vi "Fingerprint Length.vi"(8 "Error In":errorcluster) -> (0 "Error Out":errorcluster)   [LabVIEW 2017, in "Tests.lvlib" / "Session.lvlib"]
uses:
  Session.lvlib
  src/Toolkit/API/Session/API/Typedefs/Host Key Hash Types.ctl
  <vilib>/addons/_JKI Toolkits/Caraya/classes/Test/Test.lvclass
  src/Toolkit/Toolkit.lvlib
  src/Toolkit/API/Session/Session.lvclass
  <vilib>/addons/_JKI Toolkits/Caraya/classes/Assert/Assert.lvclass
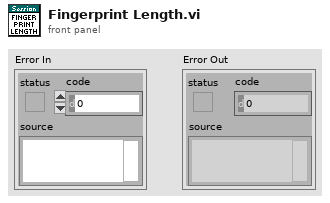
[diagram p1: front panel]
types:
  T1 = typedef "Toolkit.lvlib/Session.lvclass/Host Key Hash Types.ctl" = enum32{"MD5", "SHA1"}
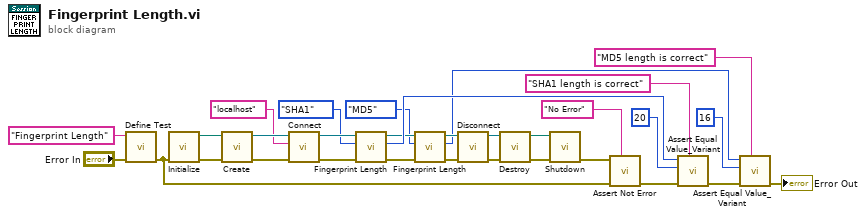
[diagram p0: block diagram]
diagram:
  n1 = call <vilib>:"Define Test.vi"("error in (no error)"="Error In", "Label (VI Title)"="Fingerprint Length") -> ("error out"=w23:errorcluster)  [unwired: 9 in]
  n2 = call "Initialize.vi"("Error In"=w23) -> ("Error Out"=w29:errorcluster, "labssh2 Shared Library Out"=w28:path)  [unwired: 9 in]
  n3 = call "Create.vi"("Error In"=w29, "labssh2 Shared Library"=w28) -> ("Error Out"=w20:errorcluster, "Sesssion"=w21:refnum<class "Session.lvclass">)  [unwired: 8 in]
  n4 = call "Connect.vi"("Error In"=w20, "Address"="localhost", "Session In"=w21) -> ("Error Out"=w12:errorcluster, "Sesssion Out"=w14:refnum<class "Session.lvclass">)  [unwired: 7 in]
  n5 = call "Fingerprint Length.vi"("Error In"=w12, "Type"=Host_Key_Hash_Types."SHA1", "Session In"=w14) -> ("Error Out"=w8:errorcluster, "Length"=w11:i32, "Sesssion Out"=w10:refnum<class "Session.lvclass">)  [unwired: 6 in]
  n6 = call "Fingerprint Length.vi"("Error In"=w8, "Type"=Host_Key_Hash_Types."MD5", "Session In"=w10) -> ("Error Out"=w7:errorcluster, "Length"=w2:i32, "Sesssion Out"=w9:refnum<class "Session.lvclass">)  [unwired: 6 in]
  n7 = call "Disconnect.vi"("Error In"=w7, "Session In"=w9) -> ("Error Out"=w17:errorcluster, "Sesssion Out"=w18:refnum<class "Session.lvclass">)  [unwired: 8 in]
  n8 = call "Destroy.vi"("Error In"=w17, "Session"=w18) -> ("Error Out"=w26:errorcluster, "labssh2 Shared Library"=w27:path)  [unwired: 8 in]
  n9 = call "Shutdown.vi"("Error In"=w26, "labssh2 Shared Library"=w27) -> ("Error Out"=w25:errorcluster)  [unwired: 9 in]
  n10 = call <vilib>:"Assert Not Error.vi"("Label"="No Error", "error in (no error)"=w23, "Not Error?"=w25) -> ("error out"=w22:errorcluster)  [unwired: 8 in]
  n11 = call <vilib>:"Assert Equal Value_Variant.vi"("Label"="SHA1 length is correct", "error in (no error)"=w22, "Y"=20 ("size(s)"), "X"=w11) -> ("error out"=w5:errorcluster)  [unwired: 7 in]
  n12 = call <vilib>:"Assert Equal Value_Variant.vi"("Label"="MD5 length is correct", "error in (no error)"=w5, "Y"=16 ("size(s)"), "X"=w2) -> ("error out"=→"Error Out":errorcluster)  [unwired: 7 in]
